vi "SLSC Enable Buttons for Online Action.vi"(8 "error in (no error)":errorcluster) -> ()   [LabVIEW 2019, in "SLSC EDS System Explorer.lvlib"]
uses:
  System Explorer/SLSC EDS System Explorer.lvlib
  <vilib>/NI VeriStand/Custom Device API/Custom Device API.lvlib
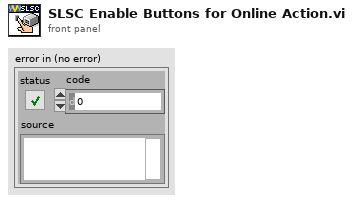
[diagram p1: front panel]
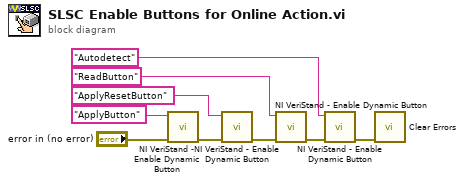
[diagram p0: block diagram]
diagram:
  n1 = call <vilib>:"NI VeriStand - Enable Dynamic Button.vi"("error in (no error)"="error in (no error)", "Button ID"="ApplyButton" ("x")) -> ("error out"=w7:errorcluster)  [unwired: 9 in]
  n2 = call <vilib>:"NI VeriStand - Enable Dynamic Button.vi"("error in (no error)"=w7, "Button ID"="ApplyResetButton" ("x")) -> ("error out"=w8:errorcluster)  [unwired: 9 in]
  n3 = call <vilib>:"NI VeriStand - Enable Dynamic Button.vi"("error in (no error)"=w8, "Button ID"="ReadButton" ("x")) -> ("error out"=w3:errorcluster)  [unwired: 9 in]
  n4 = call <vilib>:"NI VeriStand - Enable Dynamic Button.vi"("error in (no error)"=w3, "Button ID"="Autodetect") -> ("error out"=w2:errorcluster)  [unwired: 9 in]
  n5 = call <vilib>:"Clear Errors.vi"("error in (no error)"=w2) -> ()  [unwired: 1 in, 6 out]
